vi "Paths to Commands.vi"(0 "Path Properties":T3[](array[typedef]) {"Fill Orientation" items=["Horizontal", "Vertical", ""]; "Direction" items=["Forward", "Backward"]}, 1 "Path Settings":refnum<class "Path Settings.lvclass">[](array[class]), 2 "interpolation distance":dbl, 3 "paths":T7(array[cluster])) -> (5 "Lithography Data":T2(array[cluster]))   [LabVIEW 2019]
doc: "This VI processes the rectangles' data and outputs lithography data."
uses:
  <vilib>/Analysis/Matrix/Datatypes/RealMatrix.ctl
  typedefs/Path Properties - cluster.ctl
  typedefs/Voltage - cluster.ctl
  typedefs/Schedule - enum.ctl
  <userlib>/LevyLab/Relay Box/Typedefs/Resistor--enum.ctl
  Classes/Settings/Path Settings/Path Settings.lvclass
  <userlib>/LevyLab/Relay Box/Relay-Box.lvclass
  <vilib>/Analysis/Matrix/NI_Matrix.lvlib
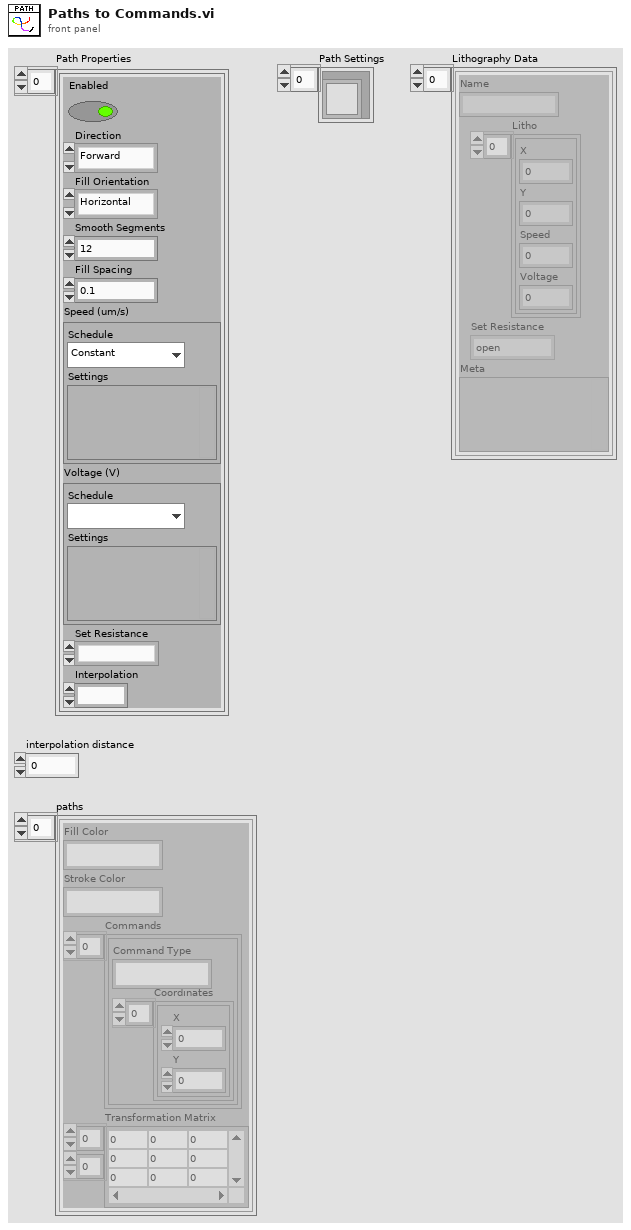
[diagram p1: front panel]
types:
  T1 = typedef "Relay-Box.lvclass/Resistor--enum.ctl" = enum16{"open", "discharge tip", "0 ohms", "100k ohm", "10M ohm", "1G ohm"}
  T2 = cluster{"Name":string, "Litho":cluster{"X":dbl, "Y":dbl, "Speed":dbl, "Voltage":dbl}[], "Set Resistance":T1, "Meta":variant}[]
  T3 = typedef "Path Properties - cluster.ctl" = cluster{"Enabled":bool, "Direction":u16, "Fill Orientation":u16, "Smooth Segments":dbl, "Fill Spacing":dbl, "Speed (um/s)":T4, "Voltage (V)":T4, "Set Resistance":T1, "Interpolation":dbl}
  T4 = typedef "Voltage - cluster.ctl" = cluster{"Schedule":T5, "Settings":variant}
  T5 = typedef "Schedule - enum.ctl" = enum16{"Constant", "Ramp", "Fn. Generator", "Formula"}
  T6 = typedef "NI_Matrix.lvlib/RealMatrix.ctl" = dbl[][]
  T7 = cluster{"Fill Color":string, "Stroke Color":string, "Commands":cluster{"Command Type":string, "Coordinates":cluster{"X":dbl, "Y":dbl}[]}[], "Transformation Matrix":T6}[]
  T8 = cluster{"Name":string, "Litho":cluster{"X":dbl, "Y":dbl, "Speed":dbl, "Voltage":dbl}[], "Set Resistance":T1}[]
  T9 = cluster{"Command Type":string, "Coordinates":cluster{"X":dbl, "Y":dbl}[]}[]
  T10 = cluster{"Horizontal X":dbl, "Horizontal X":dbl}[]
  T11 = cluster{"Name":string, "Litho":cluster{"X":dbl, "Y":dbl, "Speed":dbl, "Voltage":dbl}[], "Set Resistance":T1}
  T12 = cluster{"Name":string, "Litho":cluster{"X":dbl, "Y":dbl, "Speed":dbl, "Voltage":dbl}[]}
  T13 = cluster{"X":dbl, "Y":dbl, "Speed":dbl, "Voltage":dbl}[]
  T14 = cluster{"Name":string, "Litho":cluster{"X":dbl, "Y":dbl, "Speed":dbl, "Voltage":dbl}[], "Set Resistance":T1, "Meta":variant}
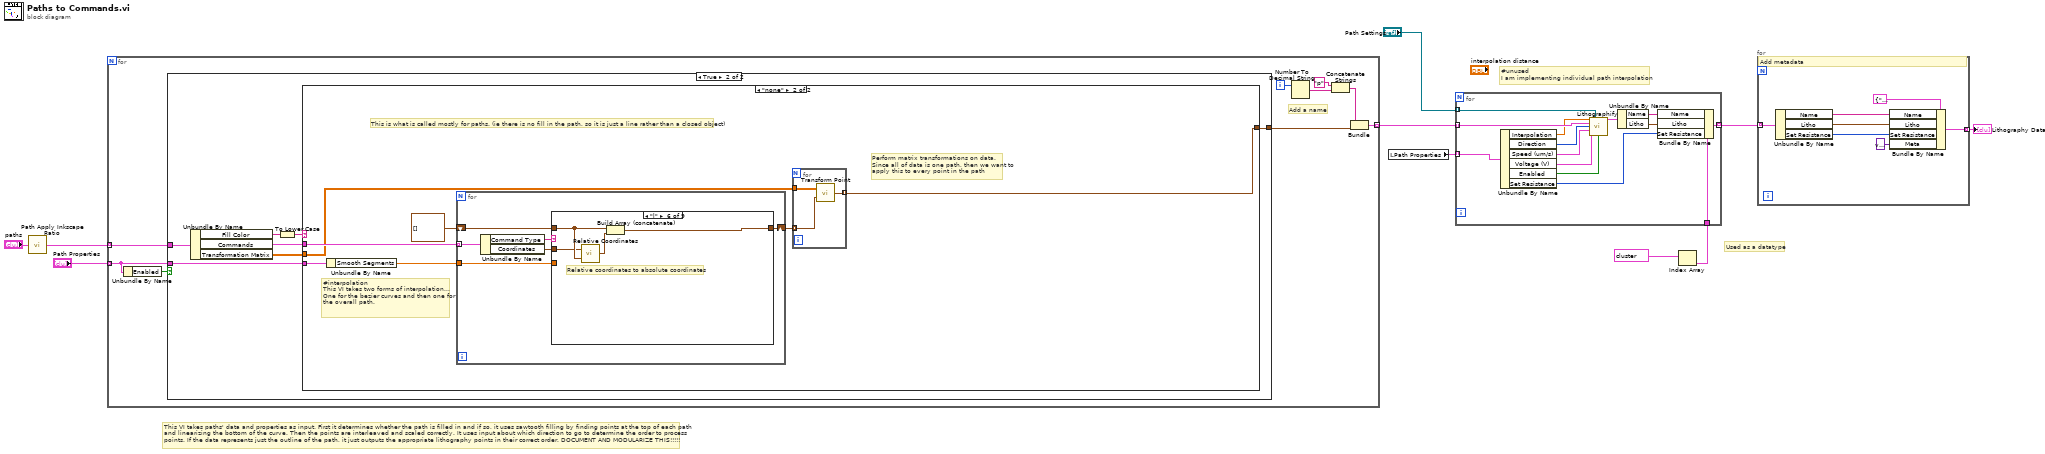
[diagram p0: block diagram]
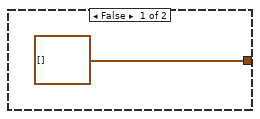
[diagram p2: hidden frame]
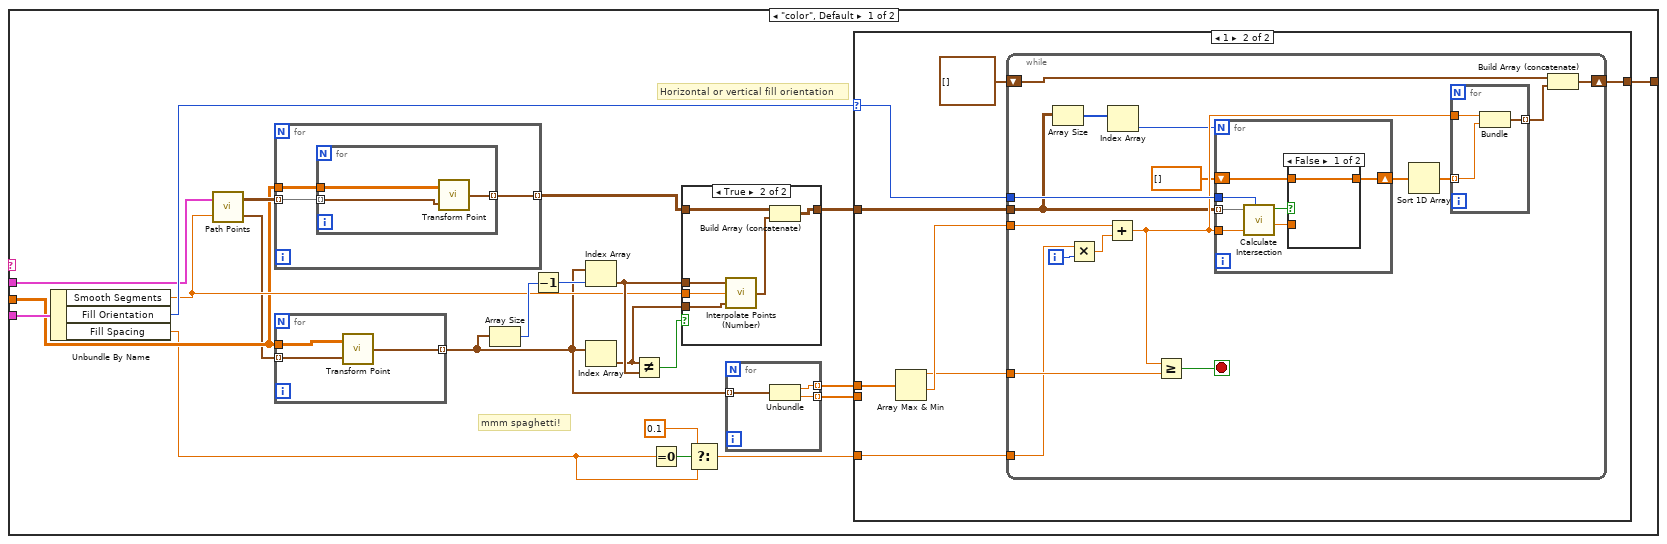
[diagram p3: hidden frame]
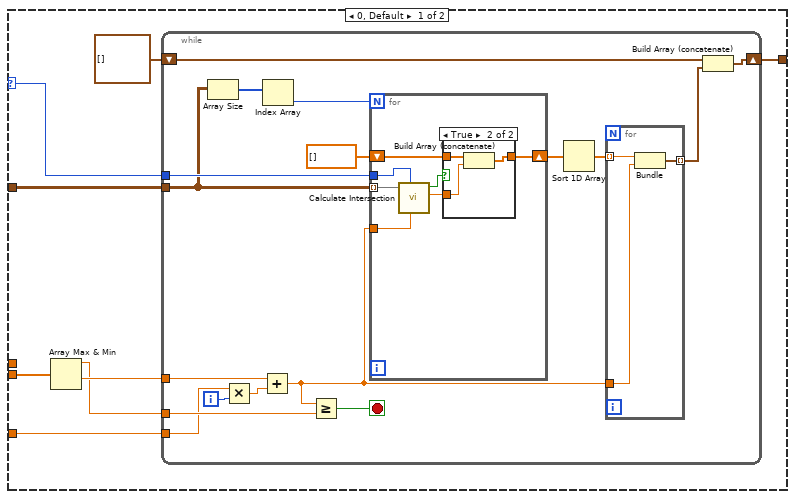
[diagram p4: hidden frame]
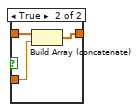
[diagram p6: hidden frame]
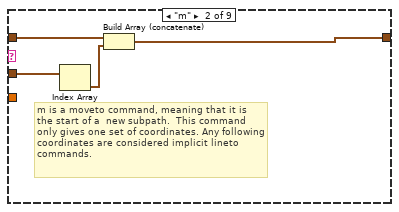
[diagram p9: hidden frame]
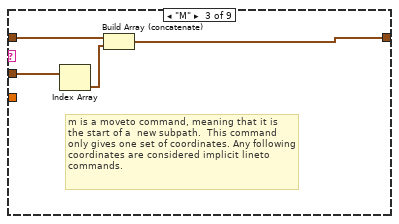
[diagram p10: hidden frame]
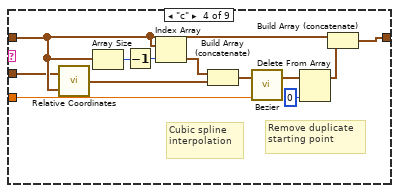
[diagram p11: hidden frame]
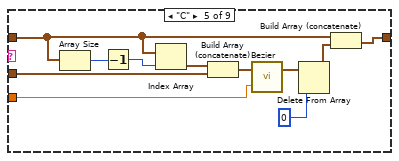
[diagram p12: hidden frame]
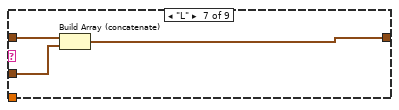
[diagram p13: hidden frame]
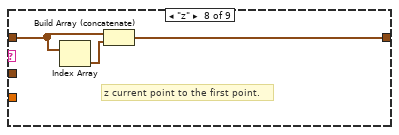
[diagram p14: hidden frame]
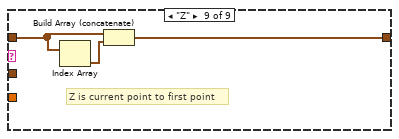
[diagram p15: hidden frame]
diagram:
  # "#unused\nI am implementing individual path interpolation"
  # "Used as a datatype"
  # "This VI takes paths' data and properties as input. First it determines whether the path is filled in and if so, it uses sawtooth filling by finding points at the top of each path \nand linearizing the bottom of the curve. Then the points are interleaved and scaled correctly. It uses input about which direction to go to determine the order to process \npoints. If the data represents just the outline of the path, it just outputs the appropriate lithography points in their correct order. DOCUMENT AND MODULARIZE THIS!!!!!"
  n1 = call "Path Apply Inkscape Ratio.vi"("paths in"="paths") -> ("paths out"=w9:T7)
  n2 = for {
    tunnel: "Path Properties" -> [w13] mode=indexing
    tunnel: [w17] -> w7 mode=indexing
    tunnel: w9 -> [w19] mode=indexing
    i -> [w14]
    # "Add a name"
    n3 = Unbundle By Name(w13) -> ("Enabled"=w12:bool)
    n4 = case shown="True" w12 {
      tunnel: w19 -> [_ w24]
      tunnel: [cluster{"X":dbl, "Y":dbl}[] [] w22] -> w18
      tunnel: w13 -> [_ w23]
      frame False {
      }
      frame True {
        n5 = Unbundle By Name(w24) -> ("Fill Color"=w27:string, "Commands"=w25:T9, "Transformation Matrix"=w21:T6)
        n6 = To Lower Case(string=w27) -> (all lower case string=w26:string)
        n7 = case shown="\"none\"" w26 {
          tunnel: w23 -> [w49 w152]
          tunnel: [w42 w148] -> w22
          tunnel: w25 -> [w38 w153]
          tunnel: w21 -> [w34 w147]
          frame "color", Default {
            # "Horizontal or vertical fill orientation"
            # "mmm spaghetti!"
            n8 = Unbundle By Name(w49) -> ("Smooth Segments"=w39:dbl, "Fill Orientation"=w45:u16, "Fill Spacing"=w29:dbl)
            n9 = call "Path Points.vi"("Smooth Segments"=w39, "Commands"=w38) -> ("Array 2"=w33:cluster{"X":dbl, "Y":dbl}[], "Array"=w36:cluster{"X":dbl, "Y":dbl}[][])
            n10 = for {
              tunnel: w36 -> [w55] mode=indexing
              tunnel: [w54] -> w35 mode=indexing
              tunnel: w34 -> [w53]
              n11 = for {
                tunnel: w55 -> [w58] mode=indexing
                tunnel: [w57] -> w54 mode=indexing
                tunnel: w53 -> [w56]
                n12 = call "Transform Point.vi"("Point to Transform"=w58, "Transformation Matrix"=w56) -> ("Transformed Point"=w57:cluster{"X":dbl, "Y":dbl})
              }
            }
            n13 = for {
              tunnel: w33 -> [w52] mode=indexing
              tunnel: [w51] -> w32 mode=indexing
              tunnel: w34 -> [w50]
              n14 = call "Transform Point.vi"("Point to Transform"=w52, "Transformation Matrix"=w50) -> ("Transformed Point"=w51:cluster{"X":dbl, "Y":dbl})
            }
            n15 = Array Size(array=w32) -> (size(s)=w48:i32)
            n16 = Decrement(x=w48) -> (x-1=w41:i32)
            n17 = Index Array(array=w32, index=w41) -> (element=w47:cluster{"X":dbl, "Y":dbl})
            n18 = Index Array(array=w32) -> (element=w46:cluster{"X":dbl, "Y":dbl})  [unwired: 1 in]
            n19 = Not Equal?(x=w46, y=w47) -> (x != y?=w37:bool)
            n20 = Equal To 0?(x=w29) -> (x = 0?=w31:bool)
            n21 = case shown="True" w37 {
              tunnel: w35 -> [w140 w143]
              tunnel: w47 -> [_ w145]
              tunnel: w46 -> [_ w144]
              tunnel: [w140 w146] -> w43
              tunnel: w39 -> [_ w141]
              frame False {
              }
              frame True {
                n22 = call "Interpolate Points (Number).vi"("End Point"=w144, "Number of Points"=w141, "Start Point"=w145) -> ("Output Point Array"=w142:cluster{"X":dbl, "Y":dbl}[])
                n23 = Build Array (concatenate)(w143, w142) -> (w146:cluster{"X":dbl, "Y":dbl}[][])
              }
            }
            n24 = Select(t=0.1, s=w31, f=w29) -> (s? t:f=w28:dbl)
            n25 = for {
              tunnel: w32 -> [w61] mode=indexing
              tunnel: [w60] -> w40 mode=indexing
              tunnel: [w59] -> w44 mode=indexing
              n26 = Unbundle(w61) -> ("X"=w60:dbl, "Y"=w59:dbl)
            }
            n27 = case shown="1" w45 {
              selector: w45 -> [w65 w103]
              tunnel: w44 -> [w69 _]
              tunnel: w43 -> [w66 w104]
              tunnel: [w64 w105] -> w42
              tunnel: w40 -> [_ w102]
              tunnel: w28 -> [w62 w101]
              frame 0, Default {
                n28 = Array Max & Min(array=w69) -> (max value=w67:dbl, min value=w68:dbl)  [unwired: 2 out]
                n29 = while {
                  tunnel: w68 -> [w86]
                  tunnel: w67 -> [w83]
                  tunnel: w66 -> [w74]
                  tunnel: w65 -> [w81]
                  shift-right: [w76] -> w64
                  shift-left: cluster{"Horizontal X":dbl, dbl}[] [] -> [w75]
                  tunnel: w62 -> [w70]
                  i -> [w85]
                  stop <- w82 stop-if-true
                  n30 = Array Size(array=w74) -> (size(s)=w73:i32[])
                  n31 = Multiply(x=w70, y=w85) -> (x*y=w84:dbl)
                  n32 = Add(x=w86, y=w84) -> (x+y=w78:dbl)
                  n33 = Index Array(array=w73) -> (element=w72:i32)  [unwired: 1 in]
                  n34 = Greater Or Equal?(x=w78, y=w83) -> (x >= y?=w82:bool)
                  n35 = for {
                    N: w72 -> [_]
                    tunnel: w74 -> [w96] mode=indexing
                    tunnel: w81 -> [w95]
                    tunnel: w78 -> [w94]
                    shift-right: [w91] -> w80
                    shift-left: dbl[] [] -> [w90]
                    n36 = call "Calculate Intersection.vi"("Coordinate Array"=w96, "Enum"=w95, "Horizontal Y"=w94) -> ("Intersection"=w93:bool, "Horizontal X"=w92:dbl)  [unwired: 2 in, 2 out]
                    n37 = case shown="True" w93 {
                      tunnel: w92 -> [_ w100]
                      tunnel: [w97 w99] -> w91
                      tunnel: w90 -> [w97 w98]
                      frame False {
                      }
                      frame True {
                        n38 = Build Array (concatenate)(w98, w100) -> (w99:dbl[])
                      }
                    }
                  }
                  n39 = Sort 1D Array(array=w80) -> (sorted array=w79:dbl[])
                  n40 = for {
                    tunnel: w79 -> [w89] mode=indexing
                    tunnel: w78 -> [w88]
                    tunnel: [w87] -> w77 mode=indexing
                    n41 = Bundle("Horizontal X"=w89, w88) -> (w87:cluster{"Horizontal X":dbl, dbl})  [unwired: 1 in]
                  }
                  n42 = Build Array (concatenate)(w75, w77) -> (w76:cluster{"Horizontal X":dbl, dbl}[])
                }
              }
              frame 1 {
                n43 = Array Max & Min(array=w102) -> (max value=w107:dbl, min value=w108:dbl)  [unwired: 2 out]
                n44 = while {
                  tunnel: w108 -> [w125]
                  tunnel: w107 -> [w122]
                  tunnel: w104 -> [w113]
                  tunnel: w103 -> [w120]
                  shift-right: [w115] -> w105
                  shift-left: cluster{"Horizontal X":dbl, dbl}[] [] -> [w114]
                  tunnel: w101 -> [w109]
                  i -> [w124]
                  stop <- w121 stop-if-true
                  n45 = Array Size(array=w113) -> (size(s)=w112:i32[])
                  n46 = Multiply(x=w109, y=w124) -> (x*y=w123:dbl)
                  n47 = Add(x=w125, y=w123) -> (x+y=w117:dbl)
                  n48 = Index Array(array=w112) -> (element=w111:i32)  [unwired: 1 in]
                  n49 = Greater Or Equal?(x=w117, y=w122) -> (x >= y?=w121:bool)
                  n50 = for {
                    N: w111 -> [_]
                    tunnel: w113 -> [w135] mode=indexing
                    tunnel: w120 -> [w129]
                    tunnel: w117 -> [w131]
                    shift-right: [w133] -> w119
                    shift-left: dbl[] [] -> [w132]
                    n51 = call "Calculate Intersection.vi"("Coordinate Array"=w135, "Enum"=w129, "Vertical X"=w131) -> ("Intersection"=w134:bool, "Vertical Y"=w130:dbl)  [unwired: 2 in, 2 out]
                    n52 = case shown="False" w134 {
                      tunnel: w130 -> [_ w139]
                      tunnel: [w136 w138] -> w133
                      tunnel: w132 -> [w136 w137]
                      frame False {
                      }
                      frame True {
                        n53 = Build Array (concatenate)(w137, w139) -> (w138:dbl[])
                      }
                    }
                  }
                  n54 = Sort 1D Array(array=w119) -> (sorted array=w118:dbl[])
                  n55 = for {
                    tunnel: w118 -> [w127] mode=indexing
                    tunnel: w117 -> [w126]
                    tunnel: [w128] -> w116 mode=indexing
                    n56 = Bundle(w126, "Horizontal X"=w127) -> (w128:cluster{dbl, "Horizontal X":dbl})  [unwired: 1 in]
                  }
                  n57 = Build Array (concatenate)(w114, w116) -> (w115:T10)
                }
              }
            }
          }
          frame "none" {
            # "#interpolation\nThis VI takes two forms of interpolation... One for the bezier curves and then one for the overall path."
            # "Perform matrix transformations on data. Since all of data is one path, then we want to apply this to every point in the path"
            # "This is what is called mostly for paths. (ie there is no fill in the path, so it is just a line rather than a closed object)"
            n58 = Unbundle By Name(w152) -> ("Smooth Segments"=w150:dbl)
            n59 = for {
              tunnel: w153 -> [w162] mode=indexing
              shift-right: [w158] -> w149
              shift-left: cluster{"X":dbl, "Y":dbl}[] [] -> [w159]
              tunnel: w150 -> [w157]
              n60 = Unbundle By Name(w162) -> ("Command Type"=w161:string, "Coordinates"=w160:cluster{"X":dbl, "Y":dbl}[])
              n61 = case shown="\"l\"" w161 {
                tunnel: w160 -> [_ w167 w169 w176 w187 w195 w199 _ _]
                tunnel: w159 -> [w163 w166 w170 w182 w193 w197 w201 w203 w207]
                tunnel: [w163 w164 w168 w183 w194 w196 w200 w202 w205] -> w158
                tunnel: w157 -> [_ _ _ w175 w188 _ _ _ _]
                frame "other letters", Default {
                }
                frame "m" {
                  # "m is a moveto command, meaning that it is the start of a  new subpath.  This command only gives one set of coordinates. Any following coordinates are considered implicit lineto commands."
                  n62 = Index Array(array=w167) -> (element=w165:cluster{"X":dbl, "Y":dbl})  [unwired: 1 in]
                  n63 = Build Array (concatenate)(w166, w165) -> (w164:cluster{"X":dbl, "Y":dbl}[])
                }
                frame "M" {
                  # "m is a moveto command, meaning that it is the start of a  new subpath.  This command only gives one set of coordinates. Any following coordinates are considered implicit lineto commands."
                  n64 = Index Array(array=w169) -> (element=w171:cluster{"X":dbl, "Y":dbl})  [unwired: 1 in]
                  n65 = Build Array (concatenate)(w170, w171) -> (w168:cluster{"X":dbl, "Y":dbl}[])
                }
                frame "c" {
                  # "Remove duplicate starting point"
                  # "Cubic spline interpolation"
                  n66 = call "Relative Coordinates.vi"("All Coordinates"=w182, "Command Coordinates"=w176) -> ("Adjusted Command Coordinates"=w180:cluster{"X":dbl, "Y":dbl}[])
                  n67 = Array Size(array=w182) -> (size(s)=w178:i32)
                  n68 = Decrement(x=w178) -> (x-1=w177:i32)
                  n69 = Index Array(array=w182, index=w177) -> (element=w181:cluster{"X":dbl, "Y":dbl})
                  n70 = Build Array (concatenate)(w181, w180) -> (w179:cluster{"X":dbl, "Y":dbl}[])
                  n71 = call "Bezier.vi"("Segments"=w175, "Parameters"=w179) -> ("Coordinate Array"=w174:cluster{"X":dbl, "Y":dbl}[])  [unwired: 1 out]
                  n72 = Delete From Array(array=w174, index=0) -> (array with subset deleted=w173:cluster{"X":dbl, "Y":dbl}[])  [unwired: 1 in, 1 out]
                  n73 = Build Array (concatenate)(w182, w173) -> (w183:cluster{"X":dbl, "Y":dbl}[])
                }
                frame "C" {
                  n74 = Array Size(array=w193) -> (size(s)=w190:i32)
                  n75 = Decrement(x=w190) -> (x-1=w189:i32)
                  n76 = Index Array(array=w193, index=w189) -> (element=w192:cluster{"X":dbl, "Y":dbl})
                  n77 = Build Array (concatenate)(w192, w187) -> (w191:cluster{"X":dbl, "Y":dbl}[])
                  n78 = call "Bezier.vi"("Segments"=w188, "Parameters"=w191) -> ("Coordinate Array"=w186:cluster{"X":dbl, "Y":dbl}[])  [unwired: 1 out]
                  n79 = Delete From Array(array=w186, index=0) -> (array with subset deleted=w185:cluster{"X":dbl, "Y":dbl}[])  [unwired: 1 in, 1 out]
                  n80 = Build Array (concatenate)(w193, w185) -> (w194:cluster{"X":dbl, "Y":dbl}[])
                }
                frame "l" {
                  # "Relative coordinates to absolute coordinates"
                  n81 = call "Relative Coordinates.vi"("All Coordinates"=w197, "Command Coordinates"=w195) -> ("Adjusted Command Coordinates"=w198:cluster{"X":dbl, "Y":dbl}[])
                  n82 = Build Array (concatenate)(w197, w198) -> (w196:cluster{"X":dbl, "Y":dbl}[])
                }
                frame "L" {
                  n83 = Build Array (concatenate)(w201, w199) -> (w200:cluster{"X":dbl, "Y":dbl}[])
                }
                frame "z" {
                  # "z current point to the first point."
                  n84 = Index Array(array=w203) -> (element=w204:cluster{"X":dbl, "Y":dbl})  [unwired: 1 in]
                  n85 = Build Array (concatenate)(w203, w204) -> (w202:cluster{"X":dbl, "Y":dbl}[])
                }
                frame "Z" {
                  # "Z is current point to first point"
                  n86 = Index Array(array=w207) -> (element=w206:cluster{"X":dbl, "Y":dbl})  [unwired: 1 in]
                  n87 = Build Array (concatenate)(w207, w206) -> (w205:cluster{"X":dbl, "Y":dbl}[])
                }
              }
            }
            n88 = for {
              tunnel: w149 -> [w156] mode=indexing
              tunnel: [w155] -> w148 mode=indexing
              tunnel: w147 -> [w154]
              n89 = call "Transform Point.vi"("Point to Transform"=w156, "Transformation Matrix"=w154) -> ("Transformed Point"=w155:cluster{"X":dbl, "Y":dbl})
            }
          }
        }
      }
    }
    n90 = Number To Decimal String(number=w14) -> (decimal integer string=w16:string)  [unwired: 1 in]
    n91 = Concatenate Strings("p" ("string"), w16) -> (w11:string)
    n92 = Bundle(w11, w18) -> (w17:cluster{string, cluster{"X":dbl, "Y":dbl}[]})  [unwired: 1 in]
  }
  n93 = local read "Path Properties"() -> (w6:T3[])
  n94 = Index Array(array=T8 data[33360B] ("Lithography Data 2")) -> (element=w4:T11)  [unwired: 1 in]
  n95 = for {
    tunnel: w6 -> [w221] mode=indexing
    tunnel: w7 -> [w220] mode=indexing
    tunnel: [w214] -> w3 mode=indexing
    tunnel: w4 -> [w213]
    tunnel: "Path Settings" -> [w208] mode=indexing
    n96 = Unbundle By Name(w221) -> ("Interpolation"=w209:dbl, "Direction"=w219:u16, "Speed (um/s)"=w218:T4, "Voltage (V)"=w210:T4, "Enabled"=w211:bool, "Set Resistance"=w212:T1)
    n97 = call "Lithographify.vi"("interpolation distance"=w209, "Path Settings.lvclass"=w208, "Data In"=w220, "Direction"=w219, "Speed (um/s)"=w218, "Voltage (V)"=w210, "Enabled"=w211) -> ("Lithography Data"=w215:T12)  [unwired: 8 in]
    n98 = Unbundle By Name(w215) -> ("Name"=w217:string, "Litho"=w216:T13)
    n99 = Bundle By Name(cluster=w213, "Name"=w217, "Litho"=w216, "Set Resistance"=w212) -> (w214:T11)
  }
  n100 = for {
    tunnel: w3 -> [w228] mode=indexing
    tunnel: [w222] -> w2 mode=indexing
    # "Add metadata"
    n101 = Unbundle By Name(w228) -> ("Name"=w226:string, "Litho"=w225:T13, "Set Resistance"=w224:T1)
    n102 = Bundle By Name(cluster=T14 {"Name"="", "Litho"=[], "Set Resistance"=enum."open", "Meta"=variant} ("Pattern Data"), "Name"=w226, "Litho"=w225, "Set Resistance"=w224, "Meta"=variant) -> (w222:T14)
  }
  "Lithography Data" <- w2
